vi "SetTetColors.vi"(6 "Photodiode":i32, 8 "error in (no error)":errorcluster, 9 "Unsorted Tet Nums":i32[](array[numeric]), 10 "WFChart Refnum":refnum<vi>, 11 "DisplayTetrodes in":refnum<class "DisplayTetrodes.lvclass">) -> (0 "error out":errorcluster, 3 "DisplayTetrodes out":refnum<class "DisplayTetrodes.lvclass">)   [LabVIEW 2010, in "DisplayTetrodes.lvclass"]
uses:
  DisplayTetrodes.lvclass
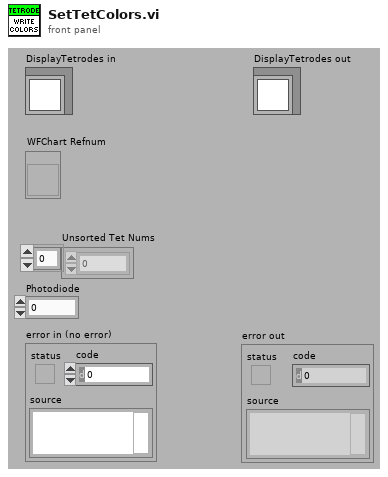
[diagram p1: front panel]
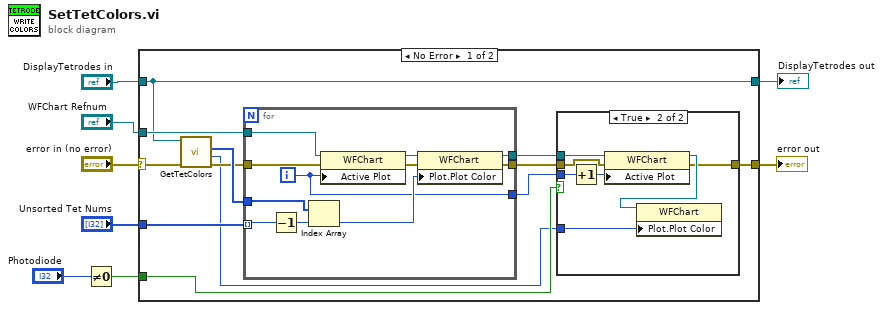
[diagram p0: block diagram]
diagram:
  n1 = Not Equal To 0?(x="Photodiode") -> (x != 0?=w1:bool)
  n2 = case shown="No Error" "error in (no error)" {
    selector: "error in (no error)" -> [w16 w41]
    tunnel: [w9 w41] -> w7
    tunnel: [w19 w40] -> w5
    tunnel: "DisplayTetrodes in" -> [w19 w40]
    tunnel: "WFChart Refnum" -> [w20 _]
    tunnel: "Unsorted Tet Nums" -> [w17 _]
    tunnel: w1 -> [w14 _]
    frame No Error {
      n3 = call-dynamic "GetTetColors.vi"("error in (no error)"=w16, "DisplayTetrodes in"=w19) -> ("error out"=w15:errorcluster, "Photodiode"=w10:u32, "Tet Colors"=w18:u32[])  [unwired: 6 in, 1 out]
      n4 = for {
        tunnel: w20 -> [w39]
        tunnel: w18 -> [w36]
        tunnel: w17 -> [w32] mode=indexing
        tunnel: w15 -> [w35]
        tunnel: [w33] -> w13
        tunnel: [w30] -> w11
        tunnel: [w29] -> w12
        i -> [w30]
        n5 = Decrement(x=w32) -> (x-1=w37:i32)
        n6 = Index Array(array=w36, index=w37) -> (element=w31:u32)
        n7 = property class="WFChart"(reference=w39, error in=w35, "Active Plot"=w30) -> (reference out=w38:refnum<vi>, error out=w34:errorcluster)
        n8 = property class="WFChart"(reference=w38, error in=w34, "Plot.Plot Color"=w31) -> (reference out=w29:refnum<vi>, error out=w33:errorcluster)
      }
      n9 = case shown="True" w14 {
        tunnel: w13 -> [w21 w23]
        tunnel: w12 -> [_ w28]
        tunnel: w11 -> [_ w26]
        tunnel: w10 -> [_ w25]
        tunnel: [w21 w22] -> w9
        frame False {
        }
        frame True {
          n10 = Increment(x=w26) -> (x+1=w27:i32)
          n11 = property class="WFChart"(reference=w28, error in=w23, "Active Plot"=w27) -> (reference out=w24:refnum<vi>, error out=w22:errorcluster)
          n12 = property class="WFChart"(reference=w24, "Plot.Plot Color"=w25) -> ()  [unwired: 1 in, 2 out]
        }
      }
    }
    frame Error {
    }
  }
  "error out" <- w7
  "DisplayTetrodes out" <- w5
